vi "Bin Pixels 8x1 (SubVI).vi"(8 "Input Valid":bool, 11 "Data In":u64) -> (0 "Output Valid":bool, 3 "Pixel Data":bool)   [LabVIEW 2015]
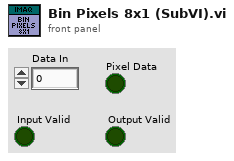
[diagram p1: front panel]
types:
  T1 = cluster{"Numeric Control":u8, "Numeric Control":u8, "Numeric Control":u8, "Numeric Control":u8, "Numeric Control":u8, "Numeric Control":u8, "Numeric Control":u8, "Numeric Control":u8}
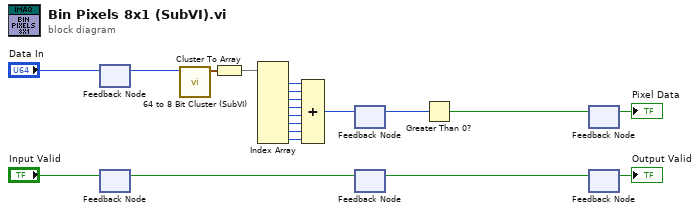
[diagram p0: block diagram]
diagram:
  n1 = feedback #1() -> (w19:u64)  [unwired: 1 in]
  n2 = feedback-in #1("Data In") -> ()
  n3 = feedback-in #2("Input Valid") -> ()
  n4 = feedback #2() -> (w10:bool)  [unwired: 1 in]
  n5 = call "64 to 8 Bit Cluster (SubVI).vi"("Data In"=w19) -> ("Data Out"=w17:T1)  [unwired: 10 in]
  n6 = Cluster To Array(cluster=w17) -> (array=w16:u8[])
  n7 = Index Array(array=w16) -> (element #1=w15:u8, element #2=w14:u8, element #3=w13:u8, element #4=w12:u8, element #5=w9:u8, element #6=w8:u8, element #7=w7:u8, element #8=w6:u8)  [unwired: 8 in]
  n8 = Compound Arithmetic op=ADD(w15, w14, w13, w12, w9, w8, w7, w6) -> (w5:u8)
  n9 = feedback-in #3(w5) -> ()
  n10 = feedback #3() -> (w4:u8)  [unwired: 1 in]
  n11 = feedback-in #4(w10) -> ()
  n12 = feedback #4() -> (w3:bool)  [unwired: 1 in]
  n13 = Greater Than 0?(x=w4) -> (x > 0?=w2:bool)
  n14 = feedback #5() -> (→"Pixel Data":bool)  [unwired: 1 in]
  n15 = feedback-in #5(w2) -> ()
  n16 = feedback #6() -> (→"Output Valid":bool)  [unwired: 1 in]
  n17 = feedback-in #6(w3) -> ()
